vi "Stop Core.vi"(10 "final error code":i32, 11 "XY Stage Process in":refnum<class "XY Stage Process.lvclass">) -> (3 "XY Stage Process out":refnum<class "XY Stage Process.lvclass">)   [LabVIEW 2022 SP3, in "XY Stage Process.lvlib" / "XY Stage Process.lvclass"]
doc: "In addition to the following, this method also sends a message to the monitor to notify it that the actor has stopped execution.\n\n(<B>Filename</B>: Actor Framework.lvlib:Actor.lvclass:Stop Core.vi)\n\nDefines what the actor does before it stops. Use the <B>final error code</B> input to determine whether the actor shut down in response to an error.\n\nBy default, this method does nothing. A descendant class may override it to define behavior, such as shutting down any processes the actor initiated in its override of the Actor Core method.\n\nCopyright: MGI\n\nAuthored by Derek Trepanier\nsupport@mooregoodideas.com\nwww.mooregoodideas.com\n\nCopyright (c) 2014, Moore Good Ideas, Inc.\n\nAll rights reserved.\n\nRedistribution and use in source and binary forms, with or without modification, are permitted provided that the following conditions are met:\n\n * Redistributions of source code must retain the above copyright notice, this list of conditions and the following disclaimer.\n * Redistributions in binary form must reproduce the above copyright notice, this list of conditions and the following disclaimer in the documentation and/or other materials provided with the distribution.\n * Neither the name of Moore Good Ideas, Inc. nor the names of its contributors may be used to endorse or promote products derived from this software without specific prior written permission.\n\nTHIS SOFTWARE IS PROVIDED BY THE COPYRIGHT HOLDERS AND CONTRIBUTORS \"AS IS\" AND ANY EXPRESS OR IMPLIED WARRANTIES, INCLUDING, BUT NOT LIMITED TO, THE IMPLIED WARRANTIES OF MERCHANTABILITY AND FITNESS FOR A PARTICULAR PURPOSE ARE DISCLAIMED. IN NO EVENT SHALL THE COPYRIGHT OWNER OR CONTRIBUTORS BE LIABLE FOR ANY DIRECT, INDIRECT, INCIDENTAL, SPECIAL, EXEMPLARY, OR CONSEQUENTIAL DAMAGES (INCLUDING, BUT NOT LIMITED TO, PROCUREMENT OF SUBSTITUTE GOODS OR SERVICES; LOSS OF USE, DATA, OR PROFITS; OR BUSINESS INTERRUPTION) HOWEVER CAUSED AND ON ANY THEORY OF LIABILITY, WHETHER IN CONTRACT, STRICT LIABILITY, OR TORT (INCLUDING NEGLIGENCE OR OTHERWISE) ARISING IN ANY WAY OUT OF THE USE OF THIS SOFTWARE, EVEN IF ADVISED OF THE POSSIBILITY OF SUCH DAMAGE."
uses:
  XY Stage Process.lvclass
  <vilib>/MGI/Monitored Actor/Monitored Actor/Monitored Actor/Monitored Actor.lvclass
  XY Stage Process.lvclass/XY Stage Process.ctl
  XY Stage Data Class/XY Stage Data Class.lvclass
  Process Framework/Process State Data/Process State Data.lvclass
  Axis Objects/iMotion Controller/iMotion Controller.lvclass
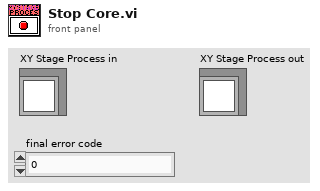
[diagram p1: front panel]
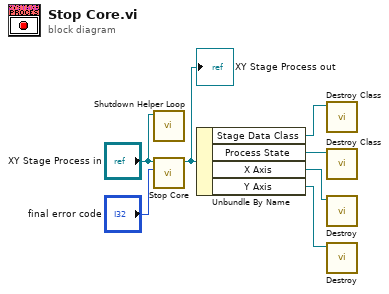
[diagram p0: block diagram]
diagram:
  n1 = call "Shutdown Helper Loop.vi"("XY Stage Process in"="XY Stage Process in") -> ()  [unwired: 11 in]
  n2 = call-parent "Stop Core.vi"("final error code"="final error code", "Monitored Actor in"="XY Stage Process in") -> ("Monitored Actor out"=w5:refnum<class "XY Stage Process.lvclass">)  [unwired: 9 in]
  "XY Stage Process out" <- w5
  n3 = Unbundle By Name(w5) -> ("Stage Data Class"=w4:refnum<data-value>, "Process State"=w3:refnum<data-value>, "X Axis"=w2:refnum<class "iMotion Controller.lvclass">, "Y Axis"=w1:refnum<class "iMotion Controller.lvclass">)
  n4 = call "Destroy Class.vi"("Stage Data Class"=w4) -> ()  [unwired: 10 in, 1 out]
  n5 = call "Destroy Class.vi"("Process State"=w3) -> ()  [unwired: 10 in, 1 out]
  n6 = call-dynamic "Destroy.vi"("Dynamic Load in"=w2) -> ()  [unwired: 9 in, 2 out]
  n7 = call-dynamic "Destroy.vi"("Dynamic Load in"=w1) -> ()  [unwired: 9 in, 2 out]
